vi "MultiVal Facade.vi"(0 "Data In":T4 {"Time" format="%<%H:%M:%S%2u>T"}, 2 "Display State In":T2, 3 "Container State":T3) -> (6 "Data Out":T4 {"Time" format="%<%H:%M:%S%2u>T"}, 7 "Display State Out":T2, 8 "Action":T1)   [LabVIEW 2013, in "Multivalue Buffer.xctl"]
uses:
  Multivalue Buffer.xctl
  MultiVal Data.ctl
  <vilib>/_xctls/Container State.ctl
  MultiVal State.ctl
  <vilib>/_xctls/Action.ctl
  <vilib>/_xctls/XControlSupport.lvlib
panel:
  out "multiVal":cluster{timestamp[], dbl[]}[](graph)
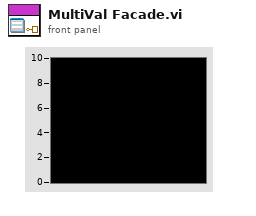
[diagram p1: front panel]
types:
  T1 = typedef "XControlSupport.lvlib/Action.ctl" = cluster{"Data Changed?":bool, "State Changed?":bool, "Action Name":string}
  T2 = typedef "Multivalue Buffer.xctl/MultiVal State.ctl" = cluster{"History":i32, "Size":cluster{"Height":i32, "Width":i32}, "axis label":string, "Graph":refnum<vi>}
  T3 = typedef "XControlSupport.lvlib/Container State.ctl" = cluster{"Indicator?":bool, "Run Mode?":bool, " Refnum":refnum<vi>}
  T4 = typedef "Multivalue Buffer.xctl/MultiVal Data.ctl" = cluster{"Time":timestamp, "Val":dbl[]}
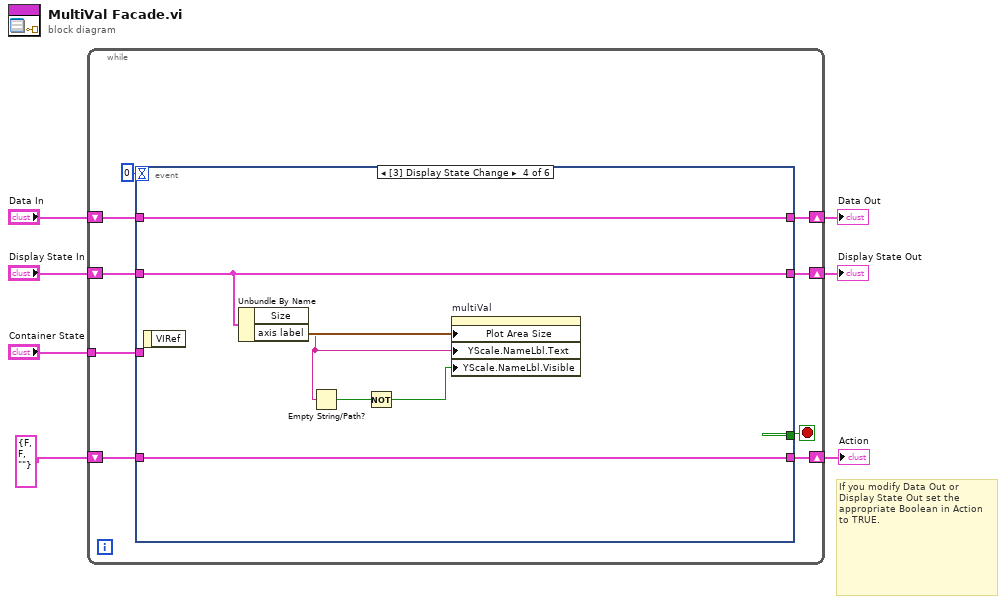
[diagram p0: block diagram]
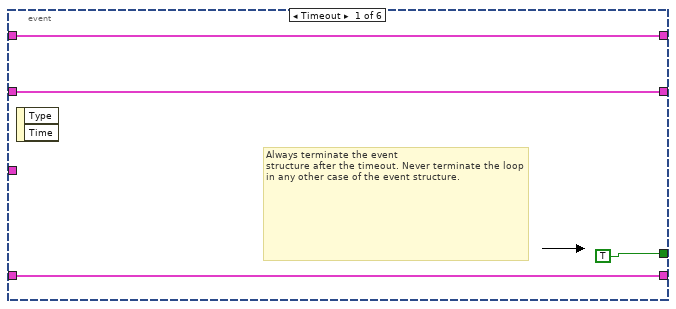
[diagram p2: hidden frame]
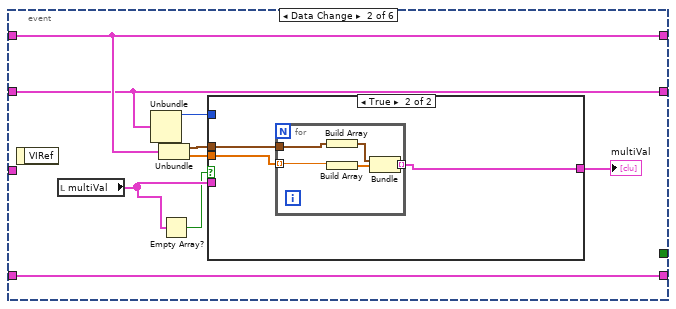
[diagram p3: hidden frame]
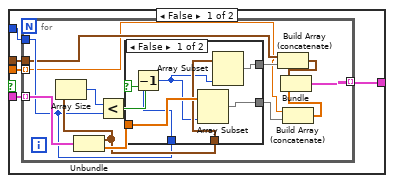
[diagram p4: hidden frame]
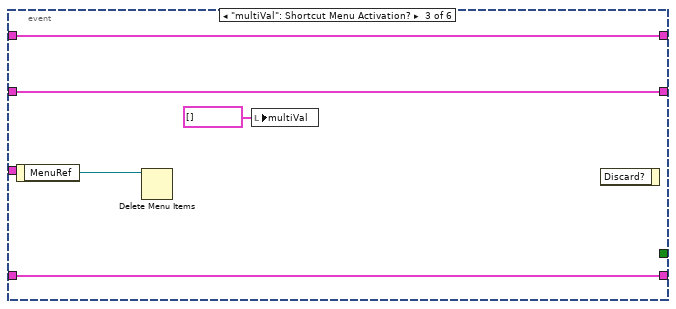
[diagram p6: hidden frame]
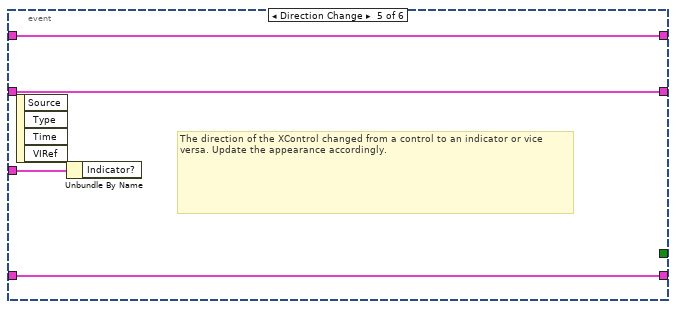
[diagram p7: hidden frame]
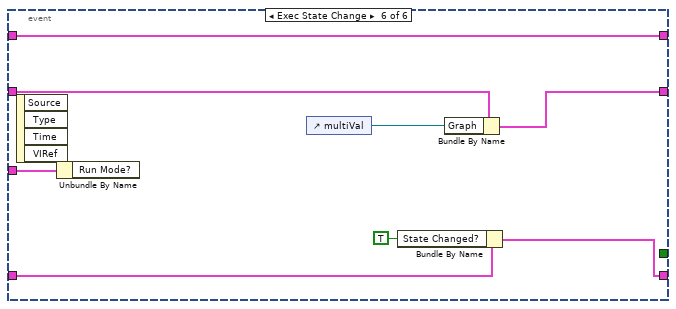
[diagram p8: hidden frame]
diagram:
  # "If you modify Data Out or\nDisplay State Out set the\nappropriate Boolean in Action\nto TRUE."
  n1 = while {
    shift-right: [w15] -> w4
    shift-left: "Display State In" -> [w16]
    tunnel: "Container State" -> [w12]
    shift-right: [w10] -> w7
    shift-left: "Data In" -> [w11]
    shift-right: [w8] -> w2
    shift-left: T1 {"Data Changed?"=FALSE, "State Changed?"=FALSE, "Action Name"=""} ("Action") -> [w9]
    stop <- w14 stop-if-true
    n2 = event shown="[3] Display State Change" {
      selector: _ -> [_ _ _ _ _ _]
      dyn-events: _ -> [_ _ _ _ _ _]
      timeout: 0 -> [_ _ _ _ _ _]
      tunnel: w16 -> [w18 w26 w68 w73 w78 w84]
      tunnel: [w18 w26 w68 w73 w78 w83] -> w15
      tunnel: [TRUE _ _ _ _ _] -> w14
      tunnel: w12 -> [_ _ _ _ w79 w87]
      tunnel: w11 -> [w17 w28 w67 w75 w77 w86]
      tunnel: [w17 w28 w67 w75 w77 w86] -> w10
      tunnel: [w19 w29 w66 w74 w76 w80] -> w8
      tunnel: w9 -> [w19 w29 w66 w74 w76 w82]
      event Timeout {
        # "Always terminate the event\nstructure after the timeout. Never terminate the loop in any other case of the event structure."
        n3 = event-data() -> ()  [unwired: 1 in, 2 out]
      }
      event Data Change {
        n4 = event-data() -> ()  [unwired: 1 in, 1 out]
        n5 = local read "multiVal"() -> (w22:cluster{timestamp[], dbl[]}[])
        n6 = Unbundle(w26) -> ("History"=w25:i32)  [unwired: 3 out]
        n7 = Unbundle(w28) -> ("Time"=w24:timestamp, "Val"=w27:dbl[])
        n8 = Empty Array?(array=w22) -> (empty?=w21:bool)
        n9 = case shown="True" w21 {
          tunnel: w27 -> [w34 w58]
          tunnel: w25 -> [w33 _]
          tunnel: w24 -> [w32 w57]
          tunnel: [w31 w56] -> w23
          tunnel: w22 -> [w30 _]
          frame False {
            n10 = for {
              tunnel: w30 -> [w46] mode=indexing
              tunnel: w34 -> [w36] mode=indexing
              tunnel: w33 -> [w41]
              tunnel: w32 -> [w39]
              tunnel: [w42] -> w31 mode=indexing
              n11 = Unbundle(w46) -> (w43:timestamp[], w44:dbl[])
              n12 = Array Size(array=w43) -> (size(s)=w47:i32)
              n13 = Less?(x=w47, y=w41) -> (x < y?=w45:bool)
              n14 = case shown="False" w45 {
                tunnel: w44 -> [w53 w54]
                tunnel: w43 -> [w51 w55]
                tunnel: w41 -> [w52 _]
                tunnel: [w49 w55] -> w40
                tunnel: [w48 w54] -> w37
                frame False {
                  n15 = Decrement(x=w52) -> (x-1=w50:i32)
                  n16 = Array Subset(array=w53, length=w50) -> (w48:dbl[])  [unwired: 1 in]
                  n17 = Array Subset(array=w51, length=w50) -> (w49:timestamp[])  [unwired: 1 in]
                }
                frame True {
                }
              }
              n18 = Build Array (concatenate)(w39, w40) -> (w38:timestamp[])
              n19 = Build Array (concatenate)(w36, w37) -> (w35:dbl[])
              n20 = Bundle(w38, w35) -> (w42:cluster{timestamp[], dbl[]})  [unwired: 1 in]
            }
          }
          frame True {
            n21 = for {
              tunnel: w58 -> [w63] mode=indexing
              tunnel: w57 -> [w62]
              tunnel: [w59] -> w56 mode=indexing
              n22 = Build Array(w62) -> (w61:timestamp[])
              n23 = Build Array(w63) -> (w60:dbl[])
              n24 = Bundle(w61, w60) -> (w59:cluster{timestamp[], dbl[]})  [unwired: 1 in]
            }
          }
        }
        "multiVal" <- w23
      }
      event "multiVal": Shortcut Menu Activation? {
        n25 = event-data() -> ("MenuRef"=w65:refnum<k9>)  [unwired: 1 in]
        n26 = Delete Menu Items(9:w65) -> ()  [unwired: 3 in, 2 out]
        n27 = local write "multiVal"(cluster{timestamp[], dbl[]}[] [] ("multiVal")) -> ()
        n28 = event-data() -> ()  [unwired: 2 in, 1 out]
      }
      event Display State Change {
        n29 = event-data() -> ()  [unwired: 1 in, 1 out]
        n30 = Unbundle By Name(w73) -> ("Size"=w72:cluster{"Height":i32, "Width":i32}, "axis label"=w71:string)
        n31 = Empty String/Path?(string/path=w71) -> (empty?=w70:bool)
        n32 = Not(x=w70) -> (.not. x?=w69:bool)
        n33 = property on="multiVal" class="XYGraph (strict)"("Plot Area Size"=w72, "YScale.NameLbl.Text"=w71, "YScale.NameLbl.Visible"=w69) -> ()  [unwired: 2 in, 2 out]
      }
      event Direction Change {
        # "The direction of the XControl changed from a control to an indicator or vice versa. Update the appearance accordingly."
        n34 = event-data() -> ()  [unwired: 1 in, 4 out]
        n35 = Unbundle By Name(w79) -> ()  [unwired: 1 out]
      }
      event Exec State Change {
        n36 = event-data() -> ()  [unwired: 1 in, 4 out]
        n37 = Unbundle By Name(w87) -> ()  [unwired: 1 out]
        n38 = control-ref of="multiVal"() -> (w85:refnum<vi>)
        n39 = Bundle By Name(cluster=w82, "State Changed?"=TRUE) -> (w80:T1)
        n40 = Bundle By Name(cluster=w84, "Graph"=w85) -> (w83:T2)
      }
    }
  }
  "Display State Out" <- w4
  "Data Out" <- w7
  "Action" <- w2
